vi "Define 1D Wave PDE (Numeric).vi"(0 "PDE in":refnum<class "NI_PDE.lvclass">, 5 "F(t, x)":dbl[][](array[numeric]), 7 "k":dbl=1.0, 9 "a":dbl, 11 "error in (no error)":errorcluster) -> (4 "PDE out":refnum<class "NI_PDE.lvclass">, 15 "error out":errorcluster)   [LabVIEW 2020, in "NI_PDE.lvlib"]
doc: "Defines the right side of a partial differential equation and its coefficients. You must manually select the polymorphic instance to use."
uses:
  <vilib>/gmath/NI_PDE.lvlib
  <vilib>/gmath/pde.llb/PDEClass/NI_PDE.lvclass
  <vilib>/gmath/pde.llb/PDEClass/PDE_Wave_1D/NI_PDE_Wave_1D.lvclass
  e:/builds/penguin/labview/branches/2020/dev/dist/vi.lib/gmath/pde.llb/PDEClass/NI_PDE.lvclass
  <vilib>/gmath/pde.llb/RHSClass/RHS_2D_Numeric/NI_RHS_2D_Numeric.lvclass
  e:/builds/penguin/labview/branches/2020/dev/dist/vi.lib/gmath/pde.llb/RHSClass/NI_RHS.lvclass
  <vilib>/gmath/pde.llb/PDEClass/PDE_2ndOrder_ConstPara/Para Data.ctl
  <vilib>/gmath/pde.llb/PDEClass/PDE_2ndOrder_ConstPara/NI_PDE_2ndOrder_ConstPara.lvclass
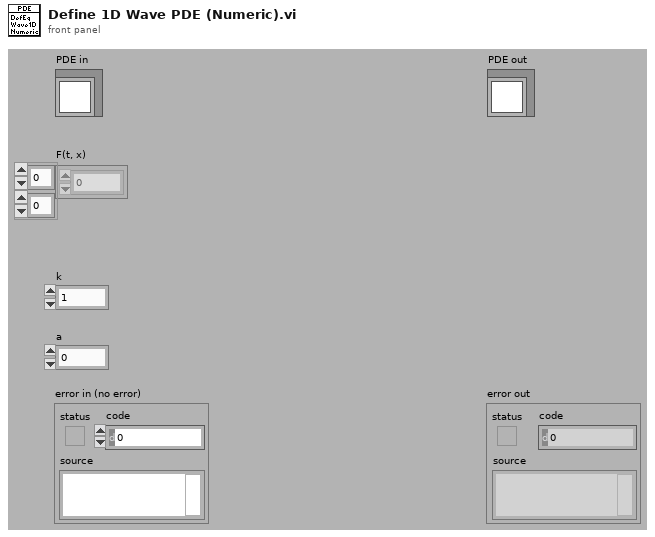
[diagram p1: front panel]
types:
  T1 = typedef "NI_PDE.lvlib/NI_PDE_2ndOrder_ConstPara.lvclass/Para Data.ctl" = cluster{"k":dbl, "a":dbl}
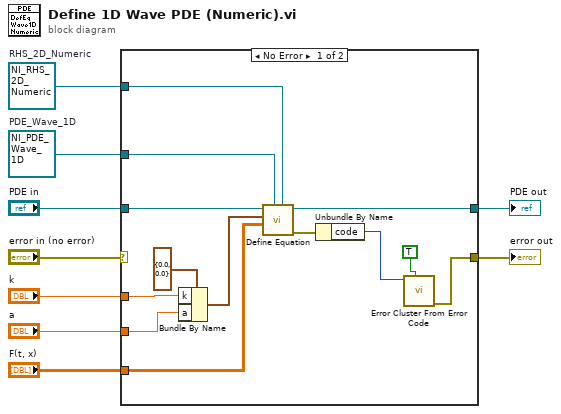
[diagram p0: block diagram]
diagram:
  w1 = refnum<class "NI_RHS_2D_Numeric.lvclass"> refnum  # RHS_2D_Numeric
  w2 = refnum<class "NI_PDE_Wave_1D.lvclass"> refnum  # PDE_Wave_1D
  n1 = case shown="No Error" "error in (no error)" {
    selector: "error in (no error)" -> [_ w24]
    tunnel: "PDE in" -> [w14 w23]
    tunnel: [w12 w23] -> w8
    tunnel: "F(t, x)" -> [w11 _]
    tunnel: "a" -> [w17 _]
    tunnel: "k" -> [w18 _]
    tunnel: [w20 w24] -> w4
    tunnel: w2 -> [w16 _]
    tunnel: w1 -> [w15 _]
    frame No Error {
      n2 = Bundle By Name(cluster=T1 {"k"=0.0, "a"=0.0} ("const para"), "k"=w18, "a"=w17) -> (w13:T1)
      n3 = call <vilib>:"Define Equation.vi"("target RHS"=w15, "target PDE"=w16, "RHS"=w11, "parameter"=w13, "PDE in"=w14) -> ("error out"=w10:errorcluster, "PDE out"=w12:refnum<class "NI_PDE.lvclass">)  [unwired: 1 in, 4 out]
      n4 = Unbundle By Name(w10) -> ("code"=w22:i32)
      n5 = call <vilib>:"Error Cluster From Error Code.vi"("show call chain? (False)"=TRUE, "error code (0)"=w22) -> ("error out"=w20:errorcluster)  [unwired: 1 in, 6 out]
    }
    frame Error {
    }
  }
  "PDE out" <- w8
  "error out" <- w4
